vi "plot_64_node.vi"() -> ()   [LabVIEW 2016]
uses:
  <vilib>/Math Plots/3D Math Plots/3D Bar/3D Bar XCtrl/3D Bar.xctl
  <vilib>/Math Plots/3D Math Plots/3D Quiver/3D Quiver XCtrl/3D Quiver.xctl
  <vilib>/Math Plots/3D Math Plots/3D Quiver/3D Quiver Datatype/Public/Plot Helper (Vector).vi
  <vilib>/Math Plots/3D Math Plots/3D Bar/3D Bar Datatype/Public/Plot Helper (Matrix).vi
  <vilib>/Math Plots/3D Math Plots/3D Bar/3D Bar Datatype/3D Bar Datatype.lvclass
  <vilib>/Math Plots/3D Math Plots/3D Quiver/3D Quiver Datatype/3D Quiver Datatype.lvclass
panel:
  out "reshaped 2":i16[][](array[numeric])
  out "3D Quiver":refnum<class "3D Plot Datatype.lvclass">[](xcontrol)
  out "3D Bar":refnum<class "3D Plot Datatype.lvclass">[](xcontrol)
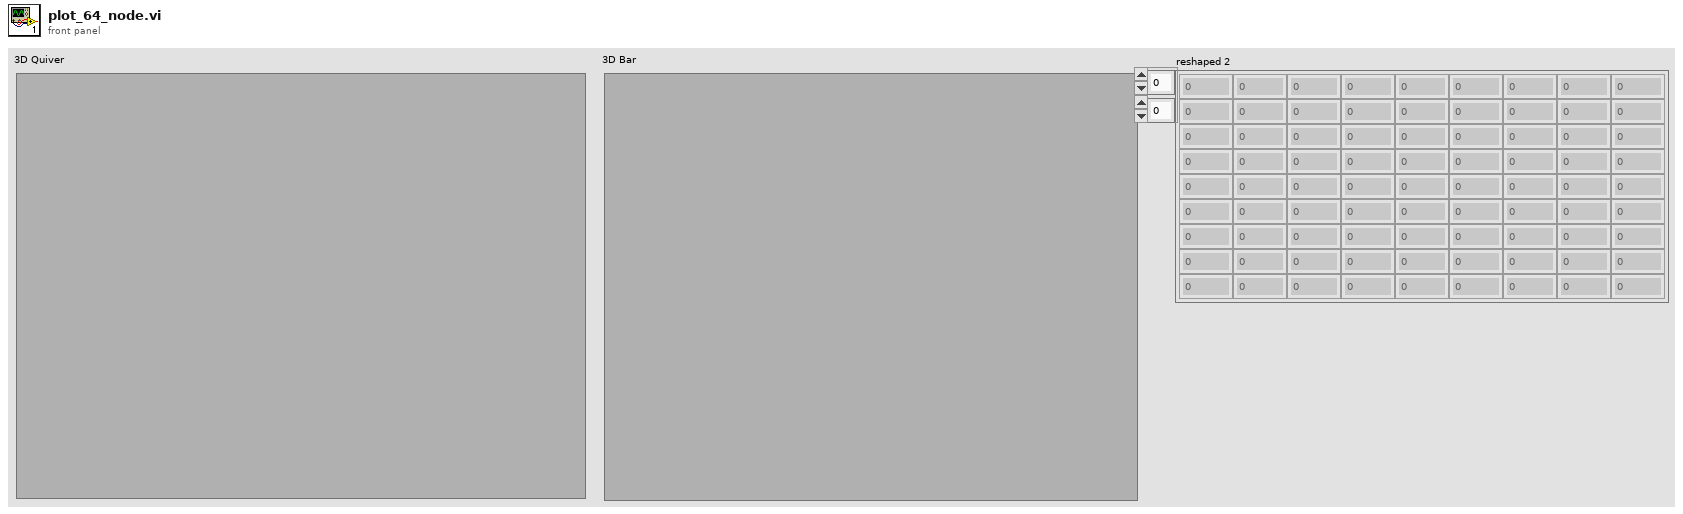
[diagram p1: front panel]
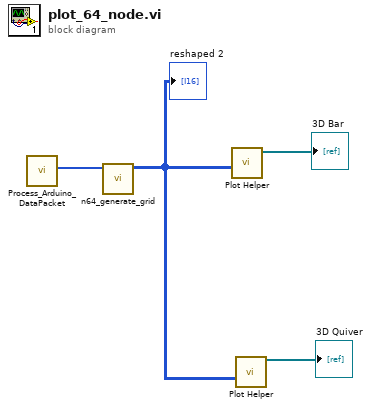
[diagram p0: block diagram]
diagram:
  n1 = call "Process_Arduino_DataPacket.vi"() -> ("Sensor Readings (Signed)"=w4:i16[])  [unwired: 8 in, 3 out]
  n2 = call "n64_generate_grid.vi"("Sensor Readings (PACKET)"=w4) -> ("Z (GRID)"=w1:i16[][])  [unwired: 8 in, 2 out]
  "reshaped 2" <- w1
  n3 = call-poly <vilib>:"Plot Helper.vi"("z matrix"=w1) -> ("3D Plot lvclass Array out"=→"3D Bar":refnum<class "3D Plot Datatype.lvclass">[])  [unwired: 2 in, 8 out]
  n4 = call-poly <vilib>:"Plot Helper.vi"("z matrix"=w1) -> ("3D Plot lvclass Array out"=→"3D Quiver":refnum<class "3D Plot Datatype.lvclass">[])  [unwired: 8 in, 6 out]
